vi "plot_usr_seq_selectableDisplay.vi"(6 "Display":u16(ring) items=["pressure", "gas flow", "vapor flow", "bias"], 10 "User-defined sequence":string[][](table)) -> (2 "Sequence Preview":cluster{dbl[], dbl[]}[](graph), 5 "seq length (hours)":dbl)   [LabVIEW 2014]
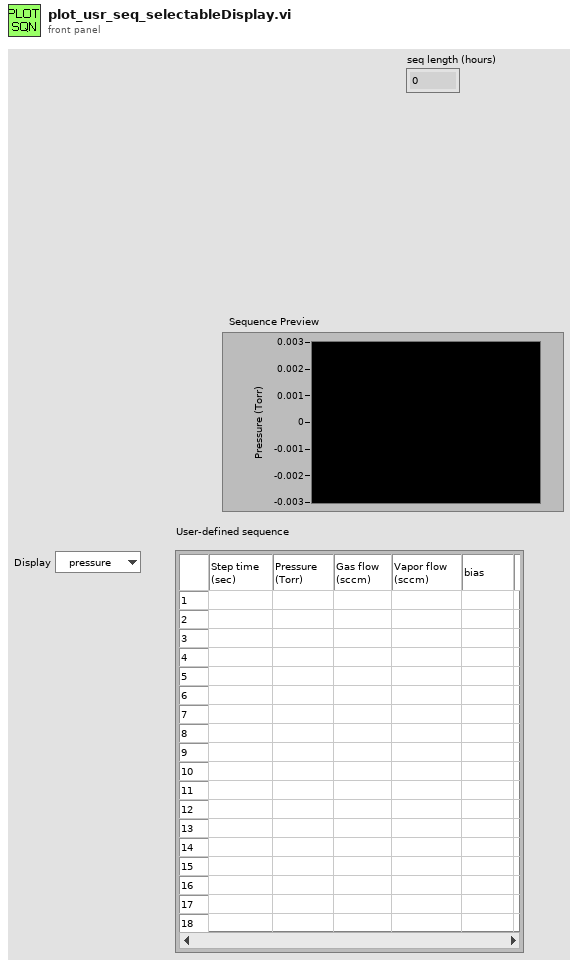
[diagram p1: front panel]
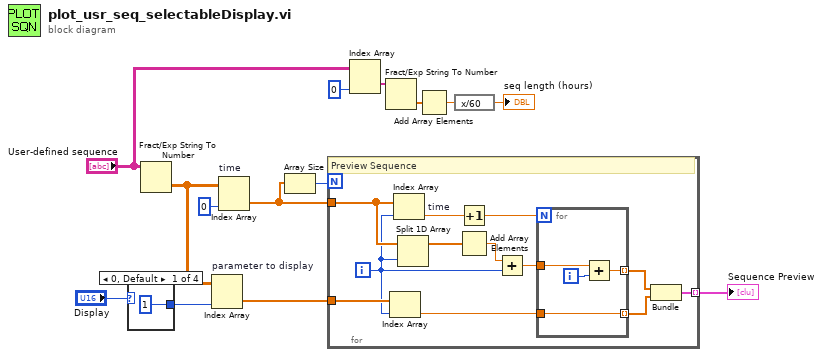
[diagram p0: block diagram]
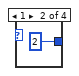
[diagram p2: hidden frame]
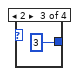
[diagram p3: hidden frame]
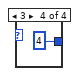
[diagram p4: hidden frame]
diagram:
  n1 = case shown="0, Default" "Display" {
    tunnel: [1 ("disabled index (col)") 2 ("disabled index (col)") 3 ("disabled index (col)") 4 ("disabled index (col)")] -> w7
    frame 0, Default {
    }
    frame 1 {
    }
    frame 2 {
    }
    frame 3 {
    }
  }
  n2 = Fract/Exp String To Number(string="User-defined sequence") -> (number=w12:dbl[][])  [unwired: 3 in, 1 out]
  n3 = Index Array "parameter to display"(array=w12, index (col)=w7) -> (element=w11:dbl[])  [unwired: 1 in]
  n4 = Index Array "time"(array=w12, index (col)=0 ("disabled index (col)")) -> (element=w9:dbl[])  [unwired: 1 in]
  n5 = Array Size(array=w9) -> (size(s)=w8:i32)
  n6 = for {
    N: w8 -> [_]
    tunnel: w9 -> [w26]
    tunnel: w11 -> [w30]
    tunnel: [w28] -> w10 mode=indexing
    i -> [w23]
    # "Preview Sequence"
    n7 = Index Array(array=w30, index=w23) -> (element=w29:dbl)
    n8 = Index Array "time"(array=w26, index=w23) -> (element=w22:dbl)
    n9 = Split 1D Array(array=w26, index=w23) -> (first subarray=w25:dbl[])  [unwired: 1 out]
    n10 = Increment(x=w22) -> (x+1=w21:dbl)
    n11 = Add Array Elements(numeric array=w25) -> (sum=w24:dbl)
    n12 = Add(x=w24, y=w23) -> (x+y=w27:dbl)
    n13 = for {
      N: w21 -> [_]
      tunnel: [w34] -> w19 mode=indexing
      tunnel: w29 -> [w34]
      tunnel: [w31] -> w20 mode=indexing
      tunnel: w27 -> [w33]
      i -> [w32]
      n14 = Add(x=w33, y=w32) -> (x+y=w31:dbl)
    }
    n15 = Bundle(w20, w19) -> (w28:cluster{dbl[], dbl[]})  [unwired: 1 in]
  }
  "Sequence Preview" <- w10
  n16 = Index Array(array="User-defined sequence", index (col)=0 ("disabled index (col)")) -> (element=w6:string[])  [unwired: 1 in]
  n17 = Fract/Exp String To Number(string=w6) -> (number=w5:dbl[])  [unwired: 3 in, 1 out]
  n18 = Add Array Elements(numeric array=w5) -> (sum=w3:dbl)
  n19 = expression code="x/60"(w3) -> (→"seq length (hours)":dbl)
